vi "RT_Control_Adrian_OnlyMicrophones.vi"(10 "rt fifo":refnum<k33>, 11 "Parameters":T1={"N_chan"=0, "Input Rate (Hz)"=0.0, "Acq Time (s)"=0.0, "NumOfWarmupIters"=0, "Size fifo"=0, "Period NCL (ms)"=0, "Timeout fifo Read"=0, "Size Sent Array"=0, "Output offsets"=[], "Input offsets"=[0.0, 0.0, 0.0, 0.0, 0.0, 0.0, 0.0, 0.0]}) -> (0 "error out":errorcluster, 2 "Delayed Cycles":dbl)   [LabVIEW 2021]
uses:
  parametersRT.ctl
  <vilib>/DAQmx/write.llb/DAQmx Write (Analog 1D DBL NChan 1Samp).vi
  <vilib>/DAQmx/read.llb/DAQmx Read (Analog 1D DBL NChan 1Samp).vi
  <vilib>/DAQmx/configure/timing.llb/DAQmx Timing (Sample Clock).vi
  <vilib>/DAQmx/miscellaneous.llb/DAQmx Fill In Error Info.vi
  <resource>/objmgr/daqmx.rc
panel:
  out "data":dbl[](array[numeric]) format="%0.2f"
  out "Numeric":i32
  out "output array":dbl[](array[numeric])
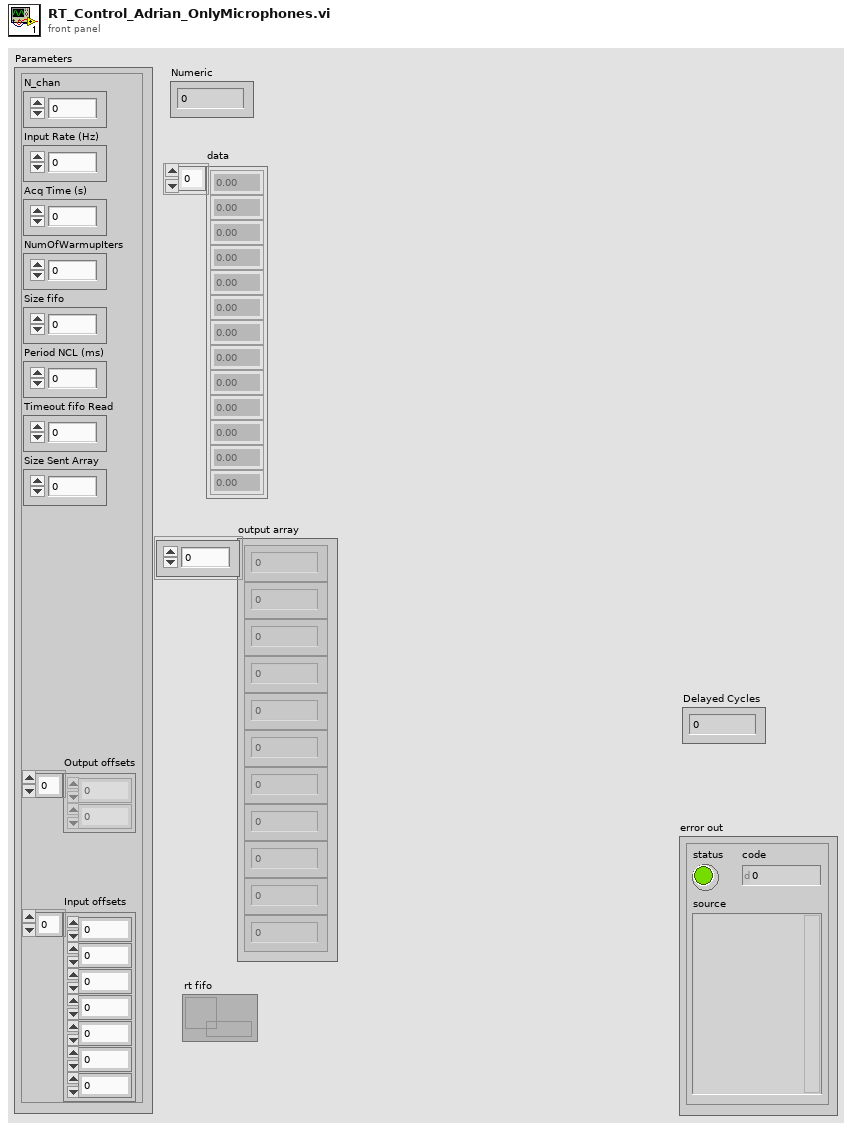
[diagram p1: front panel]
types:
  T1 = typedef "parametersRT.ctl" = cluster{"N_chan":u32, "Input Rate (Hz)":dbl, "Acq Time (s)":dbl, "NumOfWarmupIters":u32, "Size fifo":u32, "Period NCL (ms)":i64, "Timeout fifo Read":i32, "Size Sent Array":i32, "Output offsets":dbl[], "Input offsets":dbl[]}
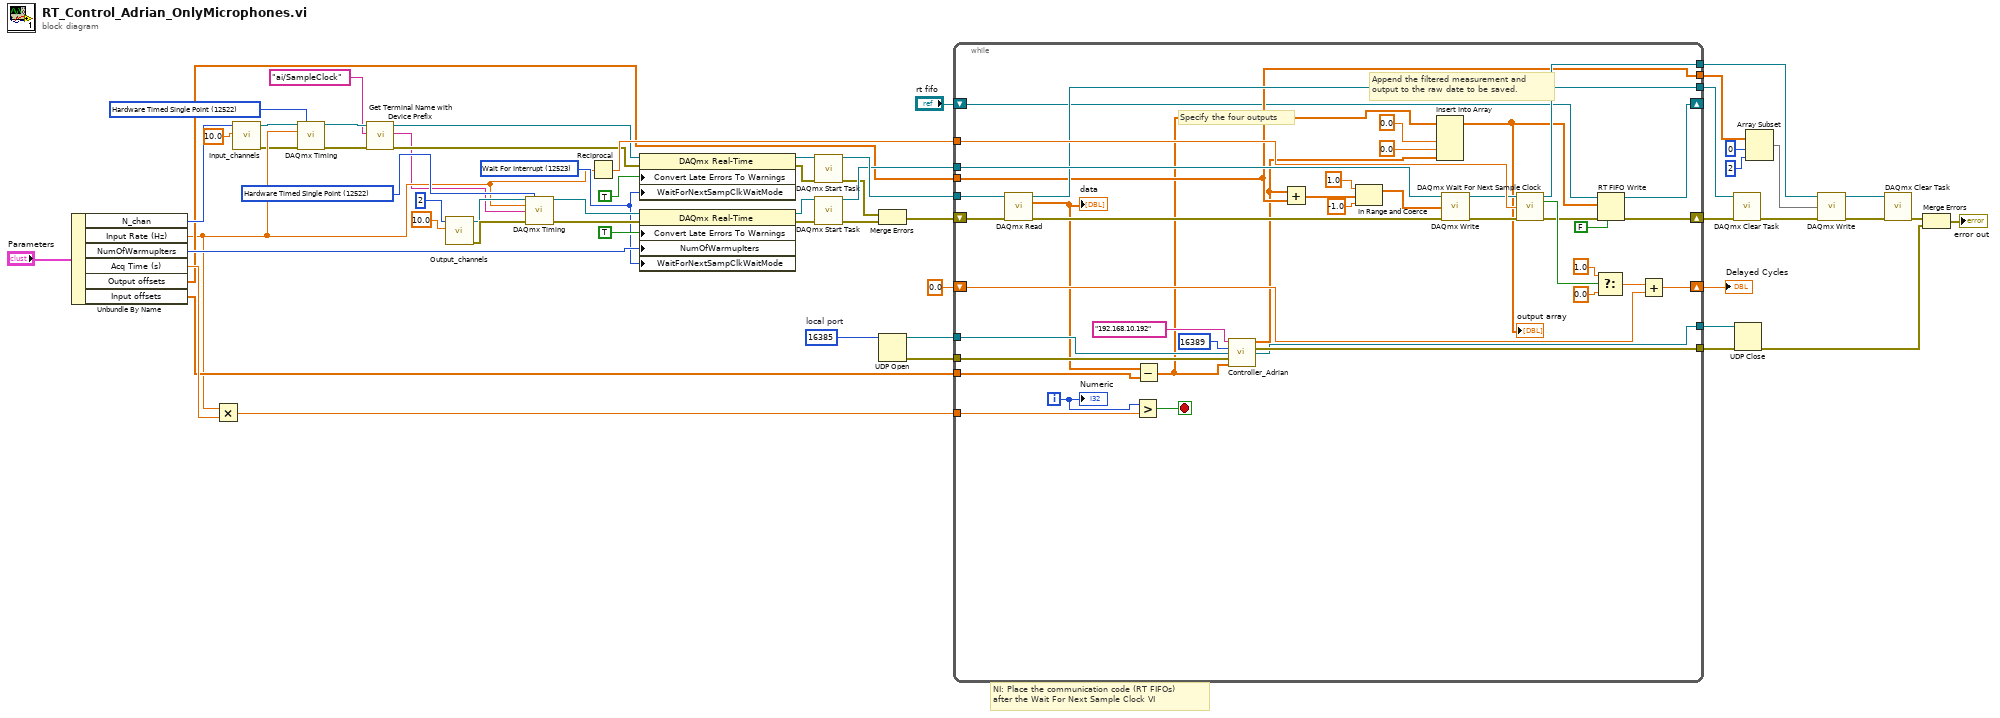
[diagram p0: block diagram]
diagram:
  w16 = u16 16385  # local port
  w23 = 12522 items=["Finite Samples"=10178, "Continuous Samples"=10123, "Hardware Timed Single Point"=12522] ("sample mode")
  w32 = 12523 items=["Wait For Interrupt"=12523, "Poll"=12524, "Yield"=12525] ("WaitForNextSampClkWaitMode")
  w58 = 12522 items=["Finite Samples"=10178, "Continuous Samples"=10123, "Hardware Timed Single Point"=12522] ("sample mode")
  # "NI: Place the communication code (RT FIFOs) \nafter the Wait For Next Sample Clock VI"
  n1 = Unbundle By Name("Parameters") -> ("N_chan"=w43:u32, "Input Rate (Hz)"=w27:dbl, "NumOfWarmupIters"=w44:u32, "Acq Time (s)"=w51:dbl, "Output offsets"=w42:dbl[], "Input offsets"=w33:dbl[])
  n2 = Multiply(x=w27, y=w51) -> (x*y=w10:dbl)
  n3 = call "Input_channels.vi"("Range"=10.0, "nchan"=w43) -> ("error out"=w25:errorcluster, "Refnum out"=w24:refnum<k21>)  [unwired: 8 in]
  n4 = call-poly <vilib>:"DAQmx Timing.vi"("task/channels in"=w24, "sample mode"=w23, "rate"=w27, "error in"=w25) -> ("task out"=w4:refnum<k21>, "error out"=w6:errorcluster)  [unwired: 10 in]
  n5 = call "Get Terminal Name with Device Prefix.vi"("error in (no error)"=w6, "Local Terminal Name"="ai/SampleClock", "task/channels in"=w4) -> ("error out"=w5:errorcluster, "Terminal Name with Device Prefix"=w2:tag, "task out"=w3:refnum<k21>)  [unwired: 6 in]
  n6 = call "Output_channels.vi"("Range"=10.0 ("Maximum Value"), "nchan"=2) -> ("error out"=w48:errorcluster, "Refnum out"=w47:refnum<k21>)  [unwired: 8 in]
  n7 = call-poly <vilib>:"DAQmx Timing.vi"("task/channels in"=w47, "sample mode"=w58, "rate"=w27, "source"=w2, "error in"=w48) -> ("task out"=w56:refnum<k21>, "error out"=w55:errorcluster)  [unwired: 9 in]
  n8 = Reciprocal(x=w27) -> (1/x=w57:dbl)
  n9 = property class="DAQmx Real-Time"(reference=w3, error in=w5, "Convert Late Errors To Warnings"=TRUE, "WaitForNextSampClkWaitMode"=w32) -> (reference out=w20:refnum<k21>, error out=w19:errorcluster)
  n10 = property class="DAQmx Real-Time"(reference=w56, error in=w55, "Convert Late Errors To Warnings"=TRUE, "NumOfWarmupIters"=w44, "WaitForNextSampClkWaitMode"=w32) -> (reference out=w52:refnum<k21>, error out=w29:errorcluster)
  n11 = call <vilib>:"DAQmx Start Task.vi"("task/channels in"=w20, "error in"=w19) -> ("task out"=w50:refnum<k21>, "error out"=w18:errorcluster)  [unwired: 12 in]
  n12 = call <vilib>:"DAQmx Start Task.vi"("task/channels in"=w52, "error in"=w29) -> ("task out"=w49:refnum<k21>, "error out"=w28:errorcluster)  [unwired: 12 in]
  n13 = Merge Errors(w18, w28) -> (w17:errorcluster)
  n14 = UDP Open(11:w16) -> (port=w14:refnum<k16>, 0:w15:errorcluster)  [unwired: 4 in, 1 out]
  n15 = while {
    shift-right: [w67] -> w26
    shift-left: w17 -> [w85]
    shift-right: [w97] -> w59
    shift-left: 0.0 ("f") -> [w72]
    tunnel: w57 -> [w95]
    tunnel: w10 -> [w93]
    tunnel: w49 -> [w91]
    tunnel: [w86] -> w53
    tunnel: w50 -> [w87]
    tunnel: [w89] -> w41
    tunnel: w42 -> [w80]
    tunnel: [w80] -> w36
    tunnel: w33 -> [w88]
    tunnel: w15 -> [w78]
    tunnel: w14 -> [w77]
    tunnel: [w76] -> w13
    tunnel: [w75] -> w12
    shift-right: [w63] -> _
    shift-left: "rt fifo" -> [w64]
    i -> [w70]
    stop <- w94 stop-if-true
    # "Append the filtered measurement and \noutput to the raw date to be saved."
    # "Specify the four outputs"
    n16 = call-poly <vilib>:"DAQmx Read.vi"("task/channels in"=w87, "error in"=w85) -> ("task out"=w86:refnum<k21>, "data"=w69:dbl[], "error out"=w84:errorcluster)  [unwired: 11 in]
    "data" <- w69
    n17 = Greater?(x=w70, y=w93) -> (0:w94:bool)
    n18 = Subtract(x=w69, y=w88) -> (x-y=w71:dbl[])
    n19 = call "Controller_Adrian.vi"("name 2"="192.168.10.192", "port or service name"=u16 16389, "connection ID"=w77, "error in (no error)"=w78, "x"=w71) -> ("*(type *) &x"=w62:dbl[], "error out"=w76:errorcluster, "connection ID out"=w75:refnum<k16>)  [unwired: 8 in]
    n20 = Add(x=w62, y=w80) -> (x+y=w82:dbl[])
    n21 = In Range and Coerce(upper limit=1.0, x=w82, lower limit=-1.0) -> (coerced(x)=w79:dbl[])  [unwired: 1 out]
    n22 = Insert Into Array(array=w71, new element #1=0.0 ("new element/subarray"), new element #2=0.0 ("new element/subarray"), new element #3=w62) -> (w65:dbl[])  [unwired: 1 in]
    "output array" <- w65
    n23 = call-poly <vilib>:"DAQmx Write.vi"("task/channels in"=w91, "data"=w79, "error in"=w84) -> ("task out"=w90:refnum<k21>, "error out"=w92:errorcluster)  [unwired: 10 in, 1 out]
    n24 = call <vilib>:"DAQmx Wait For Next Sample Clock.vi"("task/channels in"=w90, "timeout (sec)"=w95, "error in"=w92) -> ("task out"=w89:refnum<k21>, "is late?"=w96:bool, "error out"=w66:errorcluster)  [unwired: 10 in]
    n25 = Select(t=1.0, s=w96, f=0.0) -> (s? t:f=w98:dbl)
    n26 = RT FIFO Write(0:w64, 1:w65, 3:w66, 5:FALSE ("overwrite on timeout (T)")) -> (8:w63:refnum<k33>, 11:w67:errorcluster)  [unwired: 1 in, 2 out]
    n27 = Add(x=w98, y=w72) -> (x+y=w97:dbl)
    "Numeric" <- w70
  }
  "Delayed Cycles" <- w59
  n28 = call <vilib>:"DAQmx Clear Task.vi"("task in"=w53, "error in"=w26) -> ("error out"=w39:errorcluster)  [unwired: 13 in]
  n29 = UDP Close(connection ID=w12, 8:w13) -> (error out=w11:errorcluster)  [unwired: 1 out]
  n30 = Array Subset(array=w36, index=0, length=2) -> (w37:dbl[])
  n31 = call-poly <vilib>:"DAQmx Write.vi"("task/channels in"=w41, "data"=w37, "error in"=w39) -> ("task out"=w40:refnum<k21>, "error out"=w38:errorcluster)  [unwired: 10 in, 1 out]
  n32 = call <vilib>:"DAQmx Clear Task.vi"("task in"=w40, "error in"=w38) -> ("error out"=w31:errorcluster)  [unwired: 13 in]
  n33 = Merge Errors(w31, w11) -> (→"error out":errorcluster)
